vi "dfd_M-band Cosine-modulated Design Method Validation.vi"(8 "error in (no error)":errorcluster, 11 "filter bank in":T1 {"mFBank_SynthesisFilters"."mMRate_SumWl" min=1 max=32 step=1; "mFBank_SynthesisFilters"."mMRate_InputIwl" min=1 max=32 step=1; "mFBank_SynthesisFilters"."mMRate_GainWl" min=1 max=32 step=1; "mFBank_SynthesisFilters"."mMRate_OutputWl" min=1 max=32 step=1; "mFBank_SynthesisFilters"."mMRate_InputWl" min=1 max=32 step=1; "mFBank_SynthesisFilters"."mMRate_CoefWl" min=1 max=32 step=1; "mFBank_SynthesisFilters"."mMRate_Mode" items=["Default"=-1, "No Rate Change"=0, "Interpolation"=1, "Decimation"=2, "Interpolated"=3, "Rational"=4]; "mFBank_AnalysisFilters"."mMRate_SumWl" min=1 max=32 step=1; "mFBank_AnalysisFilters"."mMRate_InputIwl" min=1 max=32 step=1; "mFBank_AnalysisFilters"."mMRate_GainWl" min=1 max=32 step=1; "mFBank_AnalysisFilters"."mMRate_OutputWl" min=1 max=32 step=1; "mFBank_AnalysisFilters"."mMRate_InputWl" min=1 max=32 step=1; "mFBank_AnalysisFilters"."mMRate_CoefWl" min=1 max=32 step=1; "mFBank_AnalysisFilters"."mMRate_Mode" items=["Default"=-1, "No Rate Change"=0, "Interpolation"=1, "Decimation"=2, "Interpolated"=3, "Rational"=4]; "mFBank_Type" items=["Uniform", "Non-Uniform"]}) -> (0 "error out":errorcluster, 3 "dup filter bank":T1 {"mFBank_SynthesisFilters"."mMRate_SumWl" min=1 max=32 step=1; "mFBank_SynthesisFilters"."mMRate_InputIwl" min=1 max=32 step=1; "mFBank_SynthesisFilters"."mMRate_GainWl" min=1 max=32 step=1; "mFBank_SynthesisFilters"."mMRate_OutputWl" min=1 max=32 step=1; "mFBank_SynthesisFilters"."mMRate_InputWl" min=1 max=32 step=1; "mFBank_SynthesisFilters"."mMRate_CoefWl" min=1 max=32 step=1; "mFBank_SynthesisFilters"."mMRate_Mode" items=["Default"=-1, "No Rate Change"=0, "Interpolation"=1, "Decimation"=2, "Interpolated"=3, "Rational"=4]; "mFBank_AnalysisFilters"."mMRate_SumWl" min=1 max=32 step=1; "mFBank_AnalysisFilters"."mMRate_InputIwl" min=1 max=32 step=1; "mFBank_AnalysisFilters"."mMRate_GainWl" min=1 max=32 step=1; "mFBank_AnalysisFilters"."mMRate_OutputWl" min=1 max=32 step=1; "mFBank_AnalysisFilters"."mMRate_InputWl" min=1 max=32 step=1; "mFBank_AnalysisFilters"."mMRate_CoefWl" min=1 max=32 step=1; "mFBank_AnalysisFilters"."mMRate_Mode" items=["Default"=-1, "No Rate Change"=0, "Interpolation"=1, "Decimation"=2, "Interpolated"=3, "Rational"=4]; "mFBank_Type" items=["Uniform", "Non-Uniform"]})   [LabVIEW 2017, in "NI_DigFilter_FilterBank.lvlib"]
uses:
  <vilib>/addons/Digital Filter Design/NI_DigFilter_FilterBank.lvlib
  <vilib>/addons/Digital Filter Design/FilterBank.llb/Object/DFD Filter Bank Obj.ctl
  <vilib>/addons/Digital Filter Design/_Objects.llb/DFD Multirate Filter Obj.ctl
  <vilib>/addons/Digital Filter Design/_Objects.llb/DFD Multirate Mode.ctl
  <vilib>/addons/Digital Filter Design/_Objects.llb/DFD Coef Norm Type.ctl
  <vilib>/addons/Digital Filter Design/_Objects.llb/DFD Round-off Mode.ctl
  <vilib>/addons/Digital Filter Design/_Objects.llb/DFD FXP MRate Multiply Mode.ctl
  <vilib>/addons/Digital Filter Design/FilterBank.llb/Object/DFD Filter Bank Processing Method.ctl
  <vilib>/addons/Digital Filter Design/FilterBank.llb/Object/DFD Filter Bank Type.ctl
  <vilib>/addons/Digital Filter Design/_Misc.llb/dfd_Error Handlers (Single).vi
  <vilib>/addons/Digital Filter Design/NI_DigFilterLicensed.lvlib
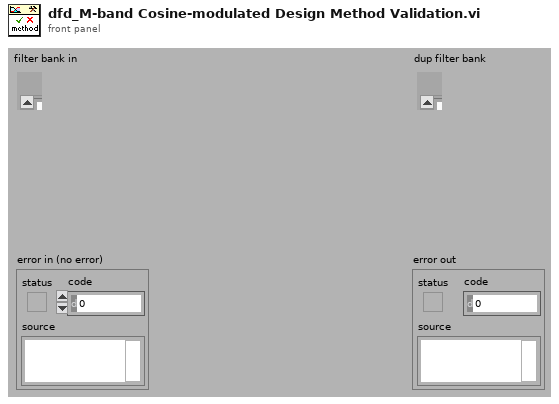
[diagram p1: front panel]
types:
  T1 = typedef "NI_DigFilter_FilterBank.lvlib/DFD Filter Bank Obj.ctl" = cluster{"mFBank_AnalysisFilters":T2[], "mFBank_SynthesisFilters":T2[], "mFBank_#Bands":i32, "mFBank_ProcMethod":T7, "mFBank_Coeffs":dbl[], "mFBank_Gain":dbl, "mFBank_Delay":i32, "mFBank_Type":T8}
  T2 = typedef "NI_DigFilterLicensed.lvlib/DFD Multirate Filter Obj.ctl" = cluster{"mMRate_Structure":enum16{"CIC", "FIR", "IIR", "Lattice"}, "mMRate_Mode":T3, "mMRate_Factor":i32, "mMRate_FIRParams":cluster{"mMRate_FIR_H":dbl[], "mMRate_FIR_IsNyquist?":bool, "mMRate_FIR_IsSymmetric?":bool}, "mMRate_CICParams":cluster{"mMRate_CIC_#Stage":i32, "mMRate_CIC_Lag":i32, "mMRate_CIC_Type":enum16{"Lowpass", "Highpass"}}, "mMRate_Order":i32, "mMRate_Version":string, "mMRate_Comments":string, "mMRate_RationalFactor":cluster{"mMRate_L":i32, "mMRate_M":i32}, "mMRate_Fs":dbl, "mMRate_Quantized?":bool, "mMRate_QFilterGain":dbl, "mMRate_CoefWl":i16, "mMRate_Scaling":cluster{"mMRate_ScaleByPowerOf2?":bool, "mMRate_ScaleType":T4}, "mMRate_InputWl":i16, "mMRate_OutputWl":i16, "mMRate_OutputMode":T5, "mMRate_MultMode":T6, "mMRate_BitPruning":bool, "mMRate_GainWl":i16, "mMRate_OutputFwl":i16, "mMRate_SumIwl":i16, "mMRate_InputIwl ":i16, "mMRate_SumWl":i16, "mMRate_CoefIwl":i16}
  T3 = typedef "NI_DigFilterLicensed.lvlib/DFD Multirate Mode.ctl" = i16
  T4 = typedef "NI_DigFilterLicensed.lvlib/DFD Coef Norm Type.ctl" = enum16{"No Norm", "Time Domain 1-Norm", "Time Domain 2-Norm", "Time Domain Inf-Norm"}
  T5 = typedef "NI_DigFilterLicensed.lvlib/DFD Round-off Mode.ctl" = enum16{"Nearest", "Truncation"}
  T6 = typedef "NI_DigFilterLicensed.lvlib/DFD FXP MRate Multiply Mode.ctl" = enum16{"Truncated", "Full"}
  T7 = typedef "NI_DigFilter_FilterBank.lvlib/DFD Filter Bank Processing Method.ctl" = enum16{"General", "2-Band QMF Lattice", "Cosine-Modulated"}
  T8 = typedef "NI_DigFilter_FilterBank.lvlib/DFD Filter Bank Type.ctl" = u16
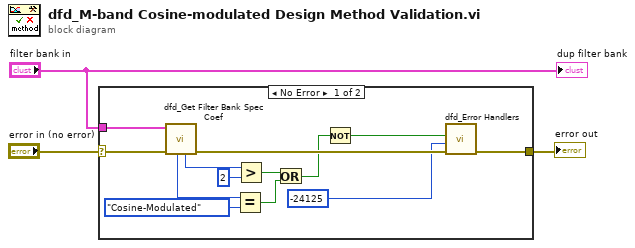
[diagram p0: block diagram]
diagram:
  n1 = case shown="No Error" "error in (no error)" {
    selector: "error in (no error)" -> [w6 w17]
    tunnel: [w16 w17] -> w3
    tunnel: "filter bank in" -> [w12 _]
    frame No Error {
      n2 = call <vilib>:"dfd_Get Filter Bank Spec Coef.vi"("error in (no error)"=w6, "filter bank"=w12) -> ("error out"=w14:errorcluster, "number of bands"=w13:i32, "processing method"=w11:T7)  [unwired: 4 in, 3 out]
      n3 = Equal?(x=w11, y=DFD_Filter_Bank_Processing_Method."Cosine-Modulated") -> (x = y?=w8:bool)
      n4 = Greater?(x=w13, y=2) -> (0:w9:bool)
      n5 = Or(x=w9, y=w8) -> (x .or. y?=w7:bool)
      n6 = Not(x=w7) -> (.not. x?=w4:bool)
      n7 = call-poly <vilib>:"dfd_Error Handlers.vi"("error in (no error)"=w14, "error code"=-24125 ("ERR_NOT_COSINE_MODULATED"), "condition failed?"=w4) -> ("error out"=w16:errorcluster)  [unwired: 8 in]
    }
    frame Error {
    }
  }
  "error out" <- w3
  "dup filter bank" <- "filter bank in"
